vi "Log to Disk.vi"(8 "error in (no error)":errorcluster) -> ()   [LabVIEW 2019, in "Logger.lvlib" / "Logger.lvclass"]
uses:
  Logger.lvclass
  Type Defs/Logging Message.ctl
  Type Defs/Logging Level.ctl
  Global Variables/Logging Configuration.vi
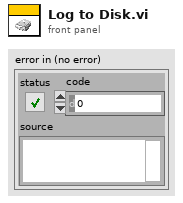
[diagram p1: front panel]
types:
  T1 = enum16{"open", "replace", "create", "open or create", "replace or create", "replace or create with confirmation"}
  T2 = typedef "Logger.lvlib/Logger.lvclass/Logging Message.ctl" = cluster{"Time Stamp":timestamp, "Logging Level":T3, "VI Name":string, "Message":string}
  T3 = typedef "Logger.lvlib/Logger.lvclass/Logging Level.ctl" = enum16{"Error", "Warning", "Info", "Trace"}
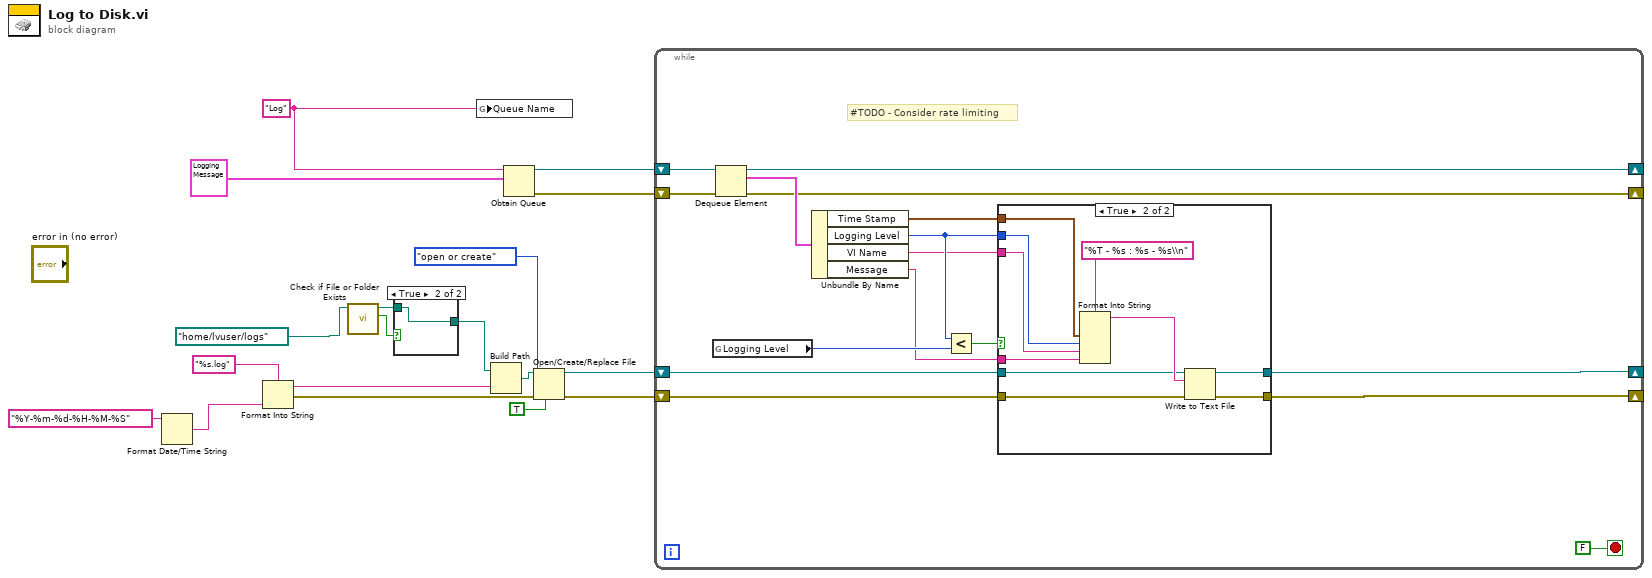
[diagram p0: block diagram]
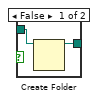
[diagram p2: hidden frame]
diagram:
  w18 = "Log" ("Queue Name")
  n1 = Format Date/Time String(time format string (%c)="%Y-%m-%d-%H-%M-%S") -> (date/time string=w3:string)  [unwired: 2 in]
  n2 = Format Into String(format string="%s.log", w3) -> (resulting string=w11:string, error out=w9:errorcluster)  [unwired: 2 in]
  n3 = call <vilib>:"Check if File or Folder Exists.vi"("path"=path "/home/lvuser/logs") -> ("file or folder exists?"=w8:bool, "dup path"=w6:path)  [unwired: 8 in, 1 out]
  n4 = case shown="True" w8 {
    tunnel: w6 -> [w20 w21]
    tunnel: [w19 w21] -> w5
    frame False {
      n5 = Create Folder(path (use dialog)=w20) -> (created path=w19:path)  [unwired: 2 in, 2 out]
    }
    frame True {
    }
  }
  n6 = global write "Logging Configuration.vi" "Queue Name"(w18) -> ()
  n7 = Build Path(base path=w5, name or relative path=w11) -> (appended path=w14:path)
  n8 = Obtain Queue(name (unnamed)=w18, element data type=T2 {"Time Stamp"=timestamp(0 s since 1904-01-01), "Logging Level"=enum."Error", "VI Name"="", "Message"=""} ("Logging Message")) -> (queue out=w16:refnum<queue>, error out=w15:errorcluster)  [unwired: 3 in, 1 out]
  n9 = Open/Create/Replace File(file path (use dialog)=w14, error in=w9, operation (0:open)=T1."open or create", disable buffering (F)=TRUE) -> (refnum out=w12:refnum<file>, error out=w13:errorcluster)  [unwired: 2 in, 1 out]
  n10 = while {
    shift-right: [w25] -> _
    shift-left: w16 -> [w37]
    shift-right: [w26] -> _
    shift-left: w15 -> [w36]
    shift-right: [w23] -> _
    shift-left: w12 -> [w27]
    shift-right: [w22] -> _
    shift-left: w13 -> [w28]
    stop <- FALSE stop-if-true
    # "#TODO - Consider rate limiting"
    n11 = global read "Logging Configuration.vi" "Logging Level"() -> (w34:T3)
    n12 = Dequeue Element(queue=w37, error in (no error)=w36) -> (queue out=w25:refnum<queue>, element=w35:T2, error out=w26:errorcluster)  [unwired: 1 in, 1 out]
    n13 = Unbundle By Name(w35) -> ("Time Stamp"=w32:timestamp, "Logging Level"=w31:T3, "VI Name"=w30:string, "Message"=w29:string)
    n14 = Less?(x=w31, y=w34) -> (x < y?=w33:bool)
    n15 = case shown="True" w33 {
      tunnel: w32 -> [_ w49]
      tunnel: w31 -> [_ w48]
      tunnel: w30 -> [_ w47]
      tunnel: w29 -> [_ w46]
      tunnel: w28 -> [w38 w43]
      tunnel: w27 -> [w39 w42]
      tunnel: [w38 w41] -> w22
      tunnel: [w39 w40] -> w23
      frame False {
      }
      frame True {
        n16 = Format Into String(format string="%T - %s : %s - %s\\n", w49, w48, w47, w46) -> (resulting string=w44:string)  [unwired: 2 in, 1 out]
        n17 = Write to Text File(file (use dialog)=w42, text=w44, error in=w43) -> (refnum out=w40:refnum<file>, error out=w41:errorcluster)  [unwired: 1 in, 1 out]
      }
    }
  }
